vi "BRig_RT__Case_Exp__State_initTrial__v3.vi"(0 "input_dataCurrent":u16[](array[numeric]), 9 "input_dataBlock":u16[][](array[numeric]), 11 "input_dataTrial":u16[][](array[numeric]), 12 "input_dataExp":u16[](array[numeric])) -> (1 "output_iTrial":u16, 2 "output_nTrial":u16, 3 "output_SolenoidReward":bool, 4 "output_dataCurrent":u16[](array[numeric]), 10 "output_dataBlock":u16[][](array[numeric]), 15 "output_dataTrial":u16[][](array[numeric]))   [LabVIEW 2014]
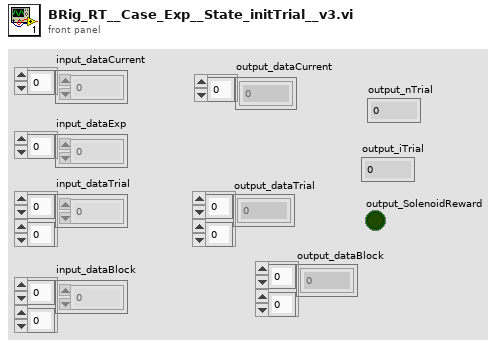
[diagram p1: front panel]
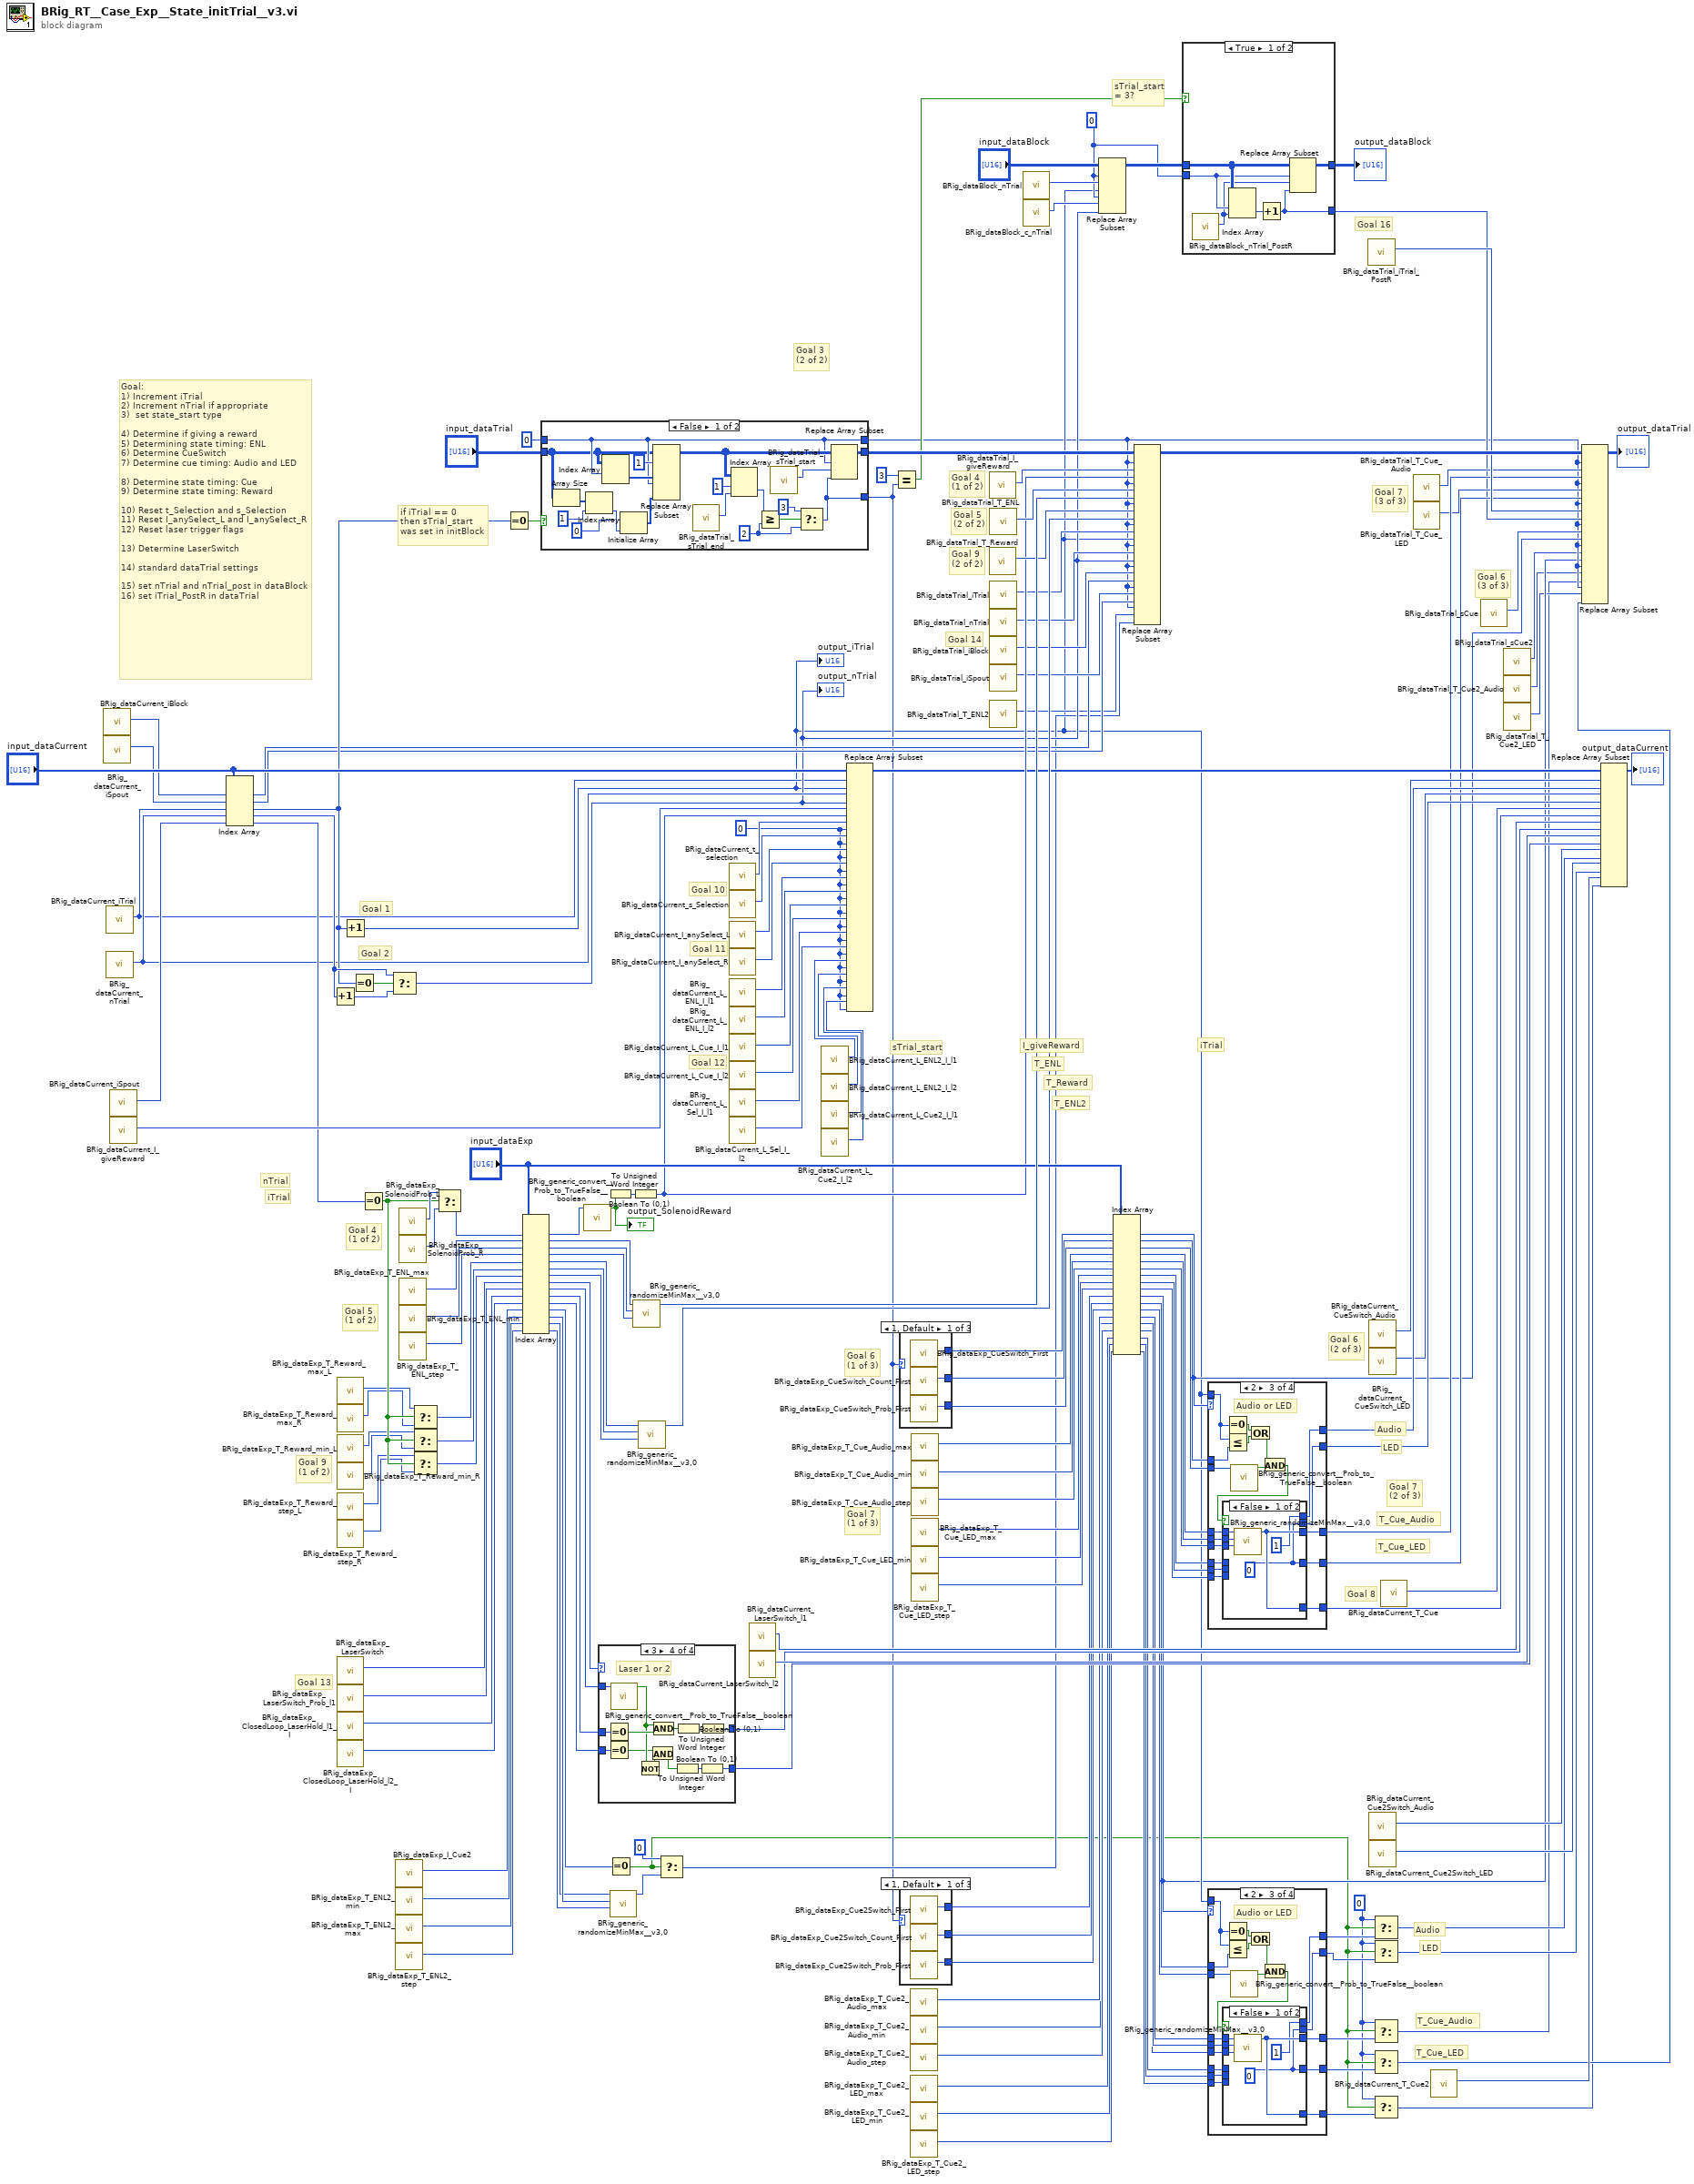
[diagram p0: block diagram]
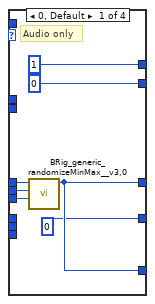
[diagram p2: hidden frame]
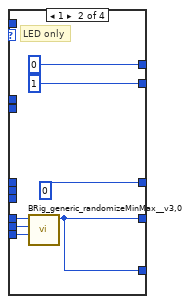
[diagram p3: hidden frame]
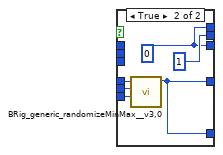
[diagram p4: hidden frame]
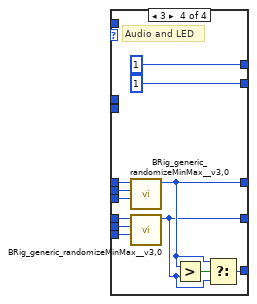
[diagram p5: hidden frame]
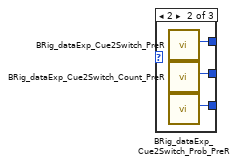
[diagram p6: hidden frame]
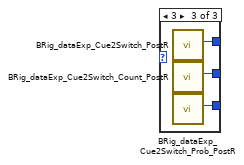
[diagram p7: hidden frame]
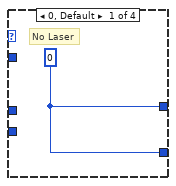
[diagram p9: hidden frame]
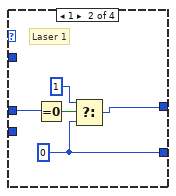
[diagram p10: hidden frame]
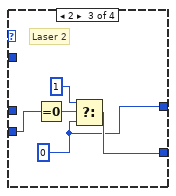
[diagram p11: hidden frame]
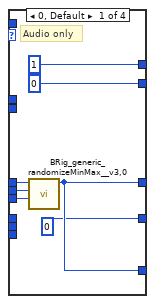
[diagram p12: hidden frame]
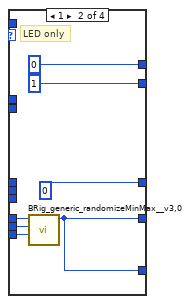
[diagram p13: hidden frame]
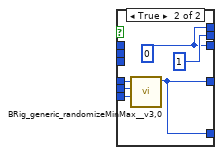
[diagram p14: hidden frame]
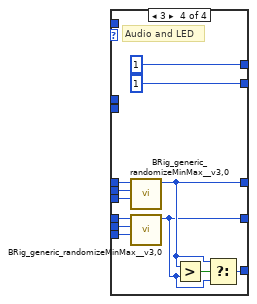
[diagram p15: hidden frame]
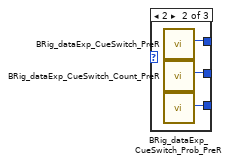
[diagram p16: hidden frame]
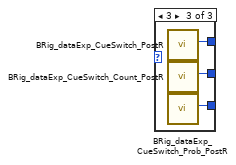
[diagram p17: hidden frame]
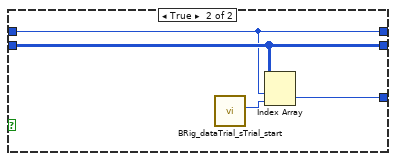
[diagram p18: hidden frame]
diagram:
  w1 = u16 0 ("t")
  w61 = 0 ("disabled index (row)")
  w40 = u16 0 ("new element/subarray")
  # "T_Cue_LED"
  # "T_Cue_Audio"
  # "LED"
  # "Audio"
  # "T_ENL2"
  # "Goal 16"
  # "Goal 6\n(3 of 3)"
  # "iTrial"
  # "sTrial_start\n= 3?"
  # "nTrial"
  # "Goal 14"
  # "Goal 13"
  # "iTrial"
  # "Goal 8"
  # "Goal 7\n(3 of 3)"
  # "Goal 7\n(2 of 3)"
  # "Goal 7\n(1 of 3)"
  # "T_Cue_LED"
  # "T_Cue_Audio"
  # "I_giveReward"
  # "Goal 4\n(1 of 2)"
  # "T_Reward"
  # "Goal 9\n(2 of 2)"
  # "Goal 9\n(1 of 2)"
  # "Goal 12"
  # "Goal 11"
  # "Goal 10"
  # "T_ENL"
  # "sTrial_start"
  # "LED"
  # "Audio"
  # "Goal 6\n(2 of 3)"
  # "Goal 6\n(1 of 3)"
  # "Goal 3\n(2 of 2)"
  # "Goal 5\n(2 of 2)"
  # "Goal 5\n(1 of 2)"
  # "Goal 4\n(1 of 2)"
  # "if iTrial == 0\nthen sTrial_start\nwas set in initBlock"
  # "Goal 2"
  # "Goal 1"
  # "Goal:\n1) Increment iTrial\n2) Increment nTrial if appropriate\n3)  set state_start type\n\n4) Determine if giving a reward\n5) Determining state timing: ENL\n6) Determine CueSwitch\n7) Determine cue timing: Audio and LED\n\n8) Determine state timing: Cue\n9) Determine state timing: Reward\n\n10) Reset t_Selection and s_Selection\n11) Reset I_anySelect_L and I_anySelect_R\n12) Reset laser trigger flags\n\n13) Determine LaserSwitch\n\n14) standard dataTrial settings\n\n15) set nTrial and nTrial_post in dataBlock\n16) set iTrial_PostR in dataTrial"
  n1 = call "BRig_dataCurrent_iBlock.vi"() -> ("output_iBlock"=w78:i32)  [unwired: 11 in]
  n2 = call "BRig_dataCurrent_iSpout.vi"() -> ("output_iSpout"=w77:i32)  [unwired: 11 in]
  n3 = call "BRig_dataCurrent_iTrial.vi"() -> ("output_iTrial"=w57:i32)  [unwired: 11 in]
  n4 = call "BRig_dataCurrent_nTrial.vi"() -> ("output_nTrial"=w59:i32)  [unwired: 11 in]
  n5 = call "BRig_dataCurrent_iSpout.vi"() -> ("output_iSpout"=w69:i32)  [unwired: 11 in]
  n6 = call "BRig_dataCurrent_I_giveReward.vi"() -> ("output_I_giveReward"=w169:i32)  [unwired: 11 in]
  n7 = Index Array(array="input_dataCurrent", index #1=w78, index #2=w77, index #3=w57, index #4=w59, index #5=w69) -> (element #1=w88:u16, element #2=w87:u16, element #3=w101:u16, element #4=w175:u16, element #5=w68:u16)
  n8 = Increment(x=w175) -> (x+1=w174:u16)
  n9 = call "BRig_dataExp_T_Reward_max_L.vi"() -> ("output_T_Reward_max_L"=w134:i32)  [unwired: 11 in]
  n10 = call "BRig_dataExp_T_Reward_max_R.vi"() -> ("output_T_Reward_max_R"=w133:i32)  [unwired: 11 in]
  n11 = call "BRig_dataExp_T_Reward_min_L.vi"() -> ("output_Tcycle_Reward_min_L"=w132:i32)  [unwired: 11 in]
  n12 = call "BRig_dataExp_T_Reward_min_R.vi"() -> ("output_T_Reward_min_R"=w131:i32)  [unwired: 11 in]
  n13 = call "BRig_dataExp_T_Reward_step_L.vi"() -> ("output_T_Reward_step_L"=w130:i32)  [unwired: 11 in]
  n14 = call "BRig_dataExp_T_Reward_step_R.vi"() -> ("output_T_Reward_step_R"=w129:i32)  [unwired: 11 in]
  n15 = call "BRig_dataExp_LaserSwitch.vi"() -> ("output_LaserSwitch"=w100:i32)  [unwired: 11 in]
  n16 = call "BRig_dataExp_LaserSwitch_Prob_l1.vi"() -> ("output_LaserSwitch_Probability_L1"=w99:i32)  [unwired: 11 in]
  n17 = call "BRig_dataExp_ClosedLoop_LaserHold_l1_I.vi"() -> ("output_CloseLoop_LaserHold_l1_I"=w74:i32)  [unwired: 11 in]
  n18 = call "BRig_dataExp_ClosedLoop_LaserHold_l2_I.vi"() -> ("output_CloseLoop_LaserHold_l2_I"=w73:i32)  [unwired: 11 in]
  n19 = Increment(x=w101) -> (x+1=w29:u16)
  "output_iTrial" <- w29
  n20 = Equal To 0?(x=w101) -> (x = 0?=w173:bool)
  n21 = Equal To 0?(x=w68) -> (x = 0?=w135:bool)
  n22 = Select(t=w175, s=w173, f=w174) -> (s? t:f=w58:u16)
  "output_nTrial" <- w58
  n23 = call "BRig_dataExp_I_Cue2.vi"() -> ("output_I_Cue2"=w56:i32)  [unwired: 11 in]
  n24 = call "BRig_dataExp_T_ENL2_min.vi"() -> ("output_T_ENL2_min"=w55:i32)  [unwired: 11 in]
  n25 = call "BRig_dataExp_T_ENL2_max.vi"() -> ("output_T_ENL2_max"=w54:i32)  [unwired: 11 in]
  n26 = call "BRig_dataExp_T_ENL2_step.vi"() -> ("output_T_ENL2_step"=w53:i32)  [unwired: 11 in]
  n27 = call "BRig_dataExp_SolenoidProb_L.vi"() -> ("output_SolenoidProbability_L"=w168:i32)  [unwired: 11 in]
  n28 = call "BRig_dataExp_SolenoidProb_R.vi"() -> ("output_SolenoidProbability_R"=w167:i32)  [unwired: 11 in]
  n29 = call "BRig_dataExp_T_ENL_max.vi"() -> ("output_T_ENL_max"=w161:i32)  [unwired: 11 in]
  n30 = call "BRig_dataExp_T_ENL_min.vi"() -> ("output_T_ENL_min"=w162:i32)  [unwired: 11 in]
  n31 = call "BRig_dataExp_T_ENL_step.vi"() -> ("output_T_ENL_step"=w163:i32)  [unwired: 11 in]
  n32 = Select(t=w134, s=w135, f=w133) -> (s? t:f=w128:i32)
  n33 = Select(t=w132, s=w135, f=w131) -> (s? t:f=w127:i32)
  n34 = Select(t=w130, s=w135, f=w129) -> (s? t:f=w126:i32)
  n35 = Select(t=w168, s=w135, f=w167) -> (s? t:f=w166:i32)
  n36 = Equal To 0?(x=w101) -> (x = 0?=w172:bool)
  n37 = Index Array(array="input_dataExp", index #1=w166, index #2=w161, index #3=w162, index #4=w163, index #5=w128, index #6=w127, index #7=w126, index #8=w100, index #9=w99, index #10=w74, index #11=w73, index #12=w56, index #13=w55, index #14=w54, index #15=w53) -> (element #1=w165:u16, element #2=w160:u16, element #3=w159:u16, element #4=w158:u16, element #5=w125:u16, element #6=w124:u16, element #7=w123:u16, element #8=w98:u16, element #9=w97:u16, element #10=w72:u16, element #11=w71:u16, element #12=w50:u16, element #13=w49:u16, element #14=w48:u16, element #15=w47:u16)
  n38 = case shown="False" w172 {
    tunnel: "input_dataTrial" -> [w182 w199]
    tunnel: [w193 w199] -> w157
    tunnel: 0 -> [w183 w198]
    tunnel: [w183 w198] -> w13
    tunnel: [w189 w196] -> w39
    frame False {
      w190 = u16 2 ("y")
      n39 = Array Size(array=w182) -> (size(s)=w181:i32[])
      n40 = Index Array(array=w181, index=1) -> (element=w179:i32)
      n41 = Index Array(array=w182, index (row)=w183) -> (element=w186:u16[])  [unwired: 1 in]
      n42 = Initialize Array(u16 0 ("index"), w179) -> (w177:u16[])
      n43 = Replace Array Subset(array=w182, new element #1=w186, index (row) #1=1 ("index (row)"), new element #2=w177, index (row) #2=w183) -> (w184:u16[][])  [unwired: 2 in]
      n44 = call "BRig_dataTrial_sTrial_end.vi"() -> ("output_sTrial_end"=w195:i32)  [unwired: 11 in]
      n45 = Index Array(array=w184, index (row)=1 ("disabled index (row)"), index (col)=w195) -> (element=w194:u16)
      n46 = Greater Or Equal?(x=w194, y=w190) -> (x >= y?=w192:bool)
      n47 = call "BRig_dataTrial_sTrial_start.vi"() -> ("output_sTrial_start"=w188:i32)  [unwired: 11 in]
      n48 = Select(t=u16 3 ("y"), s=w192, f=w190) -> (s? t:f=w189:u16)
      n49 = Replace Array Subset(array=w184, new element=w189, index (row)=w183, index (col)=w188) -> (w193:u16[][])
    }
    frame True {
      n50 = call "BRig_dataTrial_sTrial_start.vi"() -> ("output_sTrial_start"=w197:i32)  [unwired: 11 in]
      n51 = Index Array(array=w199, index (row)=w198, index (col)=w197) -> (element=w196:u16)
    }
  }
  n52 = call "BRig_generic_convert__Prob_to_TrueFalse__boolean.vi"("input_probability_u16"=w165) -> ("output_TF"=w164:bool)  [unwired: 10 in]
  "output_SolenoidReward" <- w164
  n53 = case shown="3" w98 {
    tunnel: [w200 w201 w206 w220] -> w95
    tunnel: [w200 w202 w207 w219] -> w94
    tunnel: w97 -> [_ _ _ w223]
    tunnel: w72 -> [_ w205 _ w218]
    tunnel: w71 -> [_ _ w208 w217]
    frame 0, Default {
      w200 = u16 0
      # "No Laser"
    }
    frame 1 {
      w202 = u16 0
      # "Laser 1"
      n54 = Equal To 0?(x=w205) -> (x = 0?=w204:bool)
      n55 = Select(t=u16 1, s=w204, f=w202) -> (s? t:f=w201:u16)
    }
    frame 2 {
      w206 = u16 0
      # "Laser 2"
      n56 = Equal To 0?(x=w208) -> (x = 0?=w210:bool)
      n57 = Select(t=u16 1, s=w210, f=w206) -> (s? t:f=w207:u16)
    }
    frame 3 {
      # "Laser 1 or 2"
      n58 = Equal To 0?(x=w218) -> (x = 0?=w216:bool)
      n59 = Equal To 0?(x=w217) -> (x = 0?=w212:bool)
      n60 = call "BRig_generic_convert__Prob_to_TrueFalse__boolean.vi"("input_probability_u16"=w223) -> ("output_TF"=w215:bool)  [unwired: 10 in]
      n61 = Not(x=w215) -> (.not. x?=w213:bool)
      n62 = And(x=w212, y=w213) -> (x .and. y?=w211:bool)
      n63 = And(x=w215, y=w216) -> (x .and. y?=w214:bool)
      n64 = Boolean To (0,1)(Boolean=w211) -> (0, 1=w222:i16)
      n65 = Boolean To (0,1)(Boolean=w214) -> (0, 1=w221:i16)
      n66 = To Unsigned Word Integer(number=w222) -> (unsigned 16bit integer=w219:u16)
      n67 = To Unsigned Word Integer(number=w221) -> (unsigned 16bit integer=w220:u16)
    }
  }
  n68 = Boolean To (0,1)(Boolean=w164) -> (0, 1=w176:i16)
  n69 = Equal To 0?(x=w50) -> (x = 0?=w2:bool)
  n70 = call "BRig_generic_randomizeMinMax__v3,0.vi"("Input_Increment"=w47, "Input_Min"=w49, "Input_Max"=w48) -> ("Output"=w52:u16)  [unwired: 8 in]
  n71 = To Unsigned Word Integer(number=w176) -> (unsigned 16bit integer=w119:u16)
  n72 = call "BRig_generic_randomizeMinMax__v3,0.vi"("Input_Increment"=w158, "Input_Min"=w159, "Input_Max"=w160) -> ("Output"=w155:u16)  [unwired: 8 in]
  n73 = call "BRig_generic_randomizeMinMax__v3,0.vi"("Input_Increment"=w123, "Input_Min"=w124, "Input_Max"=w125) -> ("Output"=w121:u16)  [unwired: 8 in]
  n74 = Select(t=u16 0, s=w2, f=w52) -> (s? t:f=w45:u16)
  n75 = call "BRig_dataCurrent_t_selection.vi"() -> ("output_t_selection"=w145:i32)  [unwired: 11 in]
  n76 = call "BRig_dataCurrent_s_Selection.vi"() -> ("output_s_Selection"=w144:i32)  [unwired: 11 in]
  n77 = call "BRig_dataCurrent_I_anySelect_L.vi"() -> ("output_IanySelect_L"=w143:i32)  [unwired: 11 in]
  n78 = call "BRig_dataCurrent_I_anySelect_R.vi"() -> ("output_IanySelect_R"=w142:i32)  [unwired: 11 in]
  n79 = call "BRig_dataCurrent_L_ENL_I_l1.vi"() -> ("output_L_ENL_I_l1"=w141:i32)  [unwired: 11 in]
  n80 = call "BRig_dataCurrent_L_ENL_I_l2.vi"() -> ("output_L_ENL_I_l2"=w140:i32)  [unwired: 11 in]
  n81 = call "BRig_dataCurrent_L_Cue_I_l1.vi"() -> ("output_L_Cue_I_l1"=w139:i32)  [unwired: 11 in]
  n82 = call "BRig_dataCurrent_L_Cue_I_l2.vi"() -> ("output_L_Cue_I_l2"=w138:i32)  [unwired: 11 in]
  n83 = call "BRig_dataCurrent_L_Sel_I_l1.vi"() -> ("output_L_Sel_I_l1"=w137:i32)  [unwired: 11 in]
  n84 = call "BRig_dataCurrent_L_Sel_I_l2.vi"() -> ("output_L_Sel_I_l2"=w136:i32)  [unwired: 11 in]
  n85 = call "BRig_dataCurrent_LaserSwitch_l1.vi"() -> ("output_LaserSwitch_l1"=w93:i32)  [unwired: 11 in]
  n86 = call "BRig_dataCurrent_LaserSwitch_l2.vi"() -> ("output_LaserSwitch_l2"=w96:i32)  [unwired: 11 in]
  n87 = call "BRig_dataCurrent_L_ENL2_I_l1.vi"() -> ("output_L_ENL2_I_l1"=w44:i32)  [unwired: 11 in]
  n88 = call "BRig_dataCurrent_L_ENL2_I_l2.vi"() -> ("output_L_ENL2_I_l2"=w43:i32)  [unwired: 11 in]
  n89 = call "BRig_dataCurrent_L_Cue2_I_l1.vi"() -> ("output_L_Cue2_I_l1"=w42:i32)  [unwired: 11 in]
  n90 = call "BRig_dataCurrent_L_Cue2_I_l2.vi"() -> ("output_L_Cue2_I_l2"=w41:i32)  [unwired: 11 in]
  n91 = Replace Array Subset(array="input_dataCurrent", new element #1=w29, index #1=w57, new element #2=w58, index #2=w59, new element #3=w119, index #3=w169, new element #4=w40, index #4=w145, new element #5=w40, index #5=w144, new element #6=w40, index #6=w143, new element #7=w40, index #7=w142, new element #8=w40, index #8=w141, new element #9=w40, index #9=w140, new element #10=w40, index #10=w139, new element #11=w40, index #11=w138, new element #12=w40, index #12=w137, new element #13=w40, index #13=w136, new element #14=w40, index #14=w44, new element #15=w40, index #15=w43, new element #16=w40, index #16=w42, new element #17=w40, index #17=w41) -> (w85:u16[])
  n92 = Equal?(x=u16 3 ("y"), y=w39) -> (x = y?=w62:bool)
  n93 = case shown="1, Default" w39 {
    tunnel: [w226 w227 w232] -> w152
    tunnel: [w225 w228 w231] -> w151
    tunnel: [w224 w229 w230] -> w150
    frame 1, Default {
      n94 = call "BRig_dataExp_CueSwitch_First.vi"() -> ("output_CueSwitch_First"=w226:i32)  [unwired: 11 in]
      n95 = call "BRig_dataExp_CueSwitch_Count_First.vi"() -> ("output_CueSwitch_Count_First"=w225:i32)  [unwired: 11 in]
      n96 = call "BRig_dataExp_CueSwitch_Prob_First.vi"() -> ("output_CueSwitch_Prob_First"=w224:i32)  [unwired: 11 in]
    }
    frame 2 {
      n97 = call "BRig_dataExp_CueSwitch_PreR.vi"() -> ("output_CueSwitch_PreR"=w227:i32)  [unwired: 11 in]
      n98 = call "BRig_dataExp_CueSwitch_Count_PreR.vi"() -> ("output_CueSwitch_Count_PreR"=w228:i32)  [unwired: 11 in]
      n99 = call "BRig_dataExp_CueSwitch_Prob_PreR.vi"() -> ("output_CueSwitch_Prob_PreR"=w229:i32)  [unwired: 11 in]
    }
    frame 3 {
      n100 = call "BRig_dataExp_CueSwitch_PostR.vi"() -> ("output_CueSwitch_PostR"=w232:i32)  [unwired: 11 in]
      n101 = call "BRig_dataExp_CueSwitch_Count_PostR.vi"() -> ("output_CueSwitch_Count_PostR"=w231:i32)  [unwired: 11 in]
      n102 = call "BRig_dataExp_CueSwitch_Prob_PostR.vi"() -> ("output_CueSwitch_Prob_PostR"=w230:i32)  [unwired: 11 in]
    }
  }
  n103 = case shown="1, Default" w39 {
    tunnel: [w235 w238 w241] -> w38
    tunnel: [w234 w237 w240] -> w37
    tunnel: [w233 w236 w239] -> w36
    frame 1, Default {
      n104 = call "BRig_dataExp_Cue2Switch_First.vi"() -> ("output_Cue2Switch_First"=w235:i32)  [unwired: 11 in]
      n105 = call "BRig_dataExp_Cue2Switch_Count_First.vi"() -> ("output_Cue2Switch_Count_First"=w234:i32)  [unwired: 11 in]
      n106 = call "BRig_dataExp_Cue2Switch_Prob_First.vi"() -> ("output_Cue2Switch_Prob_First"=w233:i32)  [unwired: 11 in]
    }
    frame 2 {
      n107 = call "BRig_dataExp_Cue2Switch_PreR.vi"() -> ("output_Cue2Switch_PreR"=w238:i32)  [unwired: 11 in]
      n108 = call "BRig_dataExp_Cue2Switch_Count_PreR.vi"() -> ("output_Cue2Switch_Count_PreR"=w237:i32)  [unwired: 11 in]
      n109 = call "BRig_dataExp_Cue2Switch_Prob_PreR.vi"() -> ("output_Cue2Switch_Prob_PreR"=w236:i32)  [unwired: 11 in]
    }
    frame 3 {
      n110 = call "BRig_dataExp_Cue2Switch_PostR.vi"() -> ("output_Cue2Switch_PostR"=w241:i32)  [unwired: 11 in]
      n111 = call "BRig_dataExp_Cue2Switch_Count_PostR.vi"() -> ("output_Cue2Switch_Count_PostR"=w240:i32)  [unwired: 11 in]
      n112 = call "BRig_dataExp_Cue2Switch_Prob_PostR.vi"() -> ("output_Cue2Switch_Prob_PostR"=w239:i32)  [unwired: 11 in]
    }
  }
  n113 = call "BRig_dataExp_T_Cue2_Audio_max.vi"() -> ("output_T_Cue2_Audio_max"=w35:i32)  [unwired: 11 in]
  n114 = call "BRig_dataExp_T_Cue2_Audio_min.vi"() -> ("output_T_Cue2_Audio_min"=w34:i32)  [unwired: 11 in]
  n115 = call "BRig_dataExp_T_Cue2_Audio_step.vi"() -> ("output_T_Cue2_Audio_step"=w33:i32)  [unwired: 11 in]
  n116 = call "BRig_dataExp_T_Cue2_LED_max.vi"() -> ("output_T_Cue2_LED_max"=w32:i32)  [unwired: 11 in]
  n117 = call "BRig_dataExp_T_Cue2_LED_min.vi"() -> ("output_T_Cue2_LED_min"=w31:i32)  [unwired: 11 in]
  n118 = call "BRig_dataExp_T_Cue2_LED_step.vi"() -> ("output_T_Cue2_LED_step"=w30:i32)  [unwired: 11 in]
  n119 = call "BRig_dataExp_T_Cue_Audio_max.vi"() -> ("output_T_Cue_Audio_max"=w118:i32)  [unwired: 11 in]
  n120 = call "BRig_dataExp_T_Cue_Audio_min.vi"() -> ("output_T_Cue_Audio_min"=w117:i32)  [unwired: 11 in]
  n121 = call "BRig_dataExp_T_Cue_Audio_step.vi"() -> ("output_T_Cue_Audio_step"=w116:i32)  [unwired: 11 in]
  n122 = call "BRig_dataExp_T_Cue_LED_max.vi"() -> ("output_T_Cue_LED_max"=w115:i32)  [unwired: 11 in]
  n123 = call "BRig_dataExp_T_Cue_LED_min.vi"() -> ("output_T_Cue_LED_min"=w114:i32)  [unwired: 11 in]
  n124 = call "BRig_dataExp_T_Cue_LED_step.vi"() -> ("output_T_Cue_LED_step"=w113:i32)  [unwired: 11 in]
  n125 = call "BRig_dataTrial_I_giveReward.vi"() -> ("output_I_giveReward"=w120:i32)  [unwired: 11 in]
  n126 = call "BRig_dataTrial_T_Reward.vi"() -> ("output_T_Reward"=w122:i32)  [unwired: 11 in]
  n127 = call "BRig_dataTrial_T_ENL.vi"() -> ("output_T_ENL"=w156:i32)  [unwired: 11 in]
  n128 = call "BRig_dataTrial_iTrial.vi"() -> ("output_iTrial"=w92:i32)  [unwired: 11 in]
  n129 = call "BRig_dataTrial_nTrial.vi"() -> ("output_nTrial"=w91:i32)  [unwired: 11 in]
  n130 = call "BRig_dataTrial_iBlock.vi"() -> ("output_iBlock"=w90:i32)  [unwired: 11 in]
  n131 = call "BRig_dataTrial_iSpout.vi"() -> ("output_iSpout"=w89:i32)  [unwired: 11 in]
  n132 = call "BRig_dataTrial_T_ENL2.vi"() -> ("output_T_ENL2"=w46:i32)  [unwired: 11 in]
  n133 = call "BRig_dataBlock_nTrial.vi"() -> ("output_nTrial"=w64:i32)  [unwired: 11 in]
  n134 = call "BRig_dataBlock_c_nTrial.vi"() -> ("output_c_nTrial"=w63:i32)  [unwired: 11 in]
  n135 = Replace Array Subset(array="input_dataBlock", new element #1=w29, index (row) #1=w61, index (col) #1=w64, new element #2=w58, index (row) #2=w61, index (col) #2=w63) -> (w65:u16[][])
  n136 = Index Array(array="input_dataExp", index #1=w152, index #2=w151, index #3=w150, index #4=w118, index #5=w117, index #6=w116, index #7=w115, index #8=w114, index #9=w113, index #10=w38, index #11=w37, index #12=w36, index #13=w35, index #14=w34, index #15=w33, index #16=w32, index #17=w31, index #18=w30) -> (element #1=w75:u16, element #2=w112:u16, element #3=w111:u16, element #4=w110:u16, element #5=w109:u16, element #6=w108:u16, element #7=w107:u16, element #8=w106:u16, element #9=w105:u16, element #10=w12:u16, element #11=w28:u16, element #12=w27:u16, element #13=w26:u16, element #14=w25:u16, element #15=w24:u16, element #16=w23:u16, element #17=w22:u16, element #18=w21:u16)
  n137 = Replace Array Subset(array=w157, new element #1=w119, index (row) #1=w13, index (col) #1=w120, new element #2=w155, index (row) #2=w13, index (col) #2=w156, new element #3=w121, index (row) #3=w13, index (col) #3=w122, new element #4=w29, index (row) #4=w13, index (col) #4=w92, new element #5=w58, index (row) #5=w13, index (col) #5=w91, new element #6=w88, index (row) #6=w13, index (col) #6=w90, new element #7=w87, index (row) #7=w13, index (col) #7=w89, new element #8=w45, index (row) #8=w13, index (col) #8=w46) -> (w84:u16[][])
  n138 = case shown="True" w62 {
    tunnel: w65 -> [w247 w248]
    tunnel: [w245 w248] -> w86
    tunnel: [w242 _] -> w60
    tunnel: w61 -> [w244 _]
    frame True {
      n139 = call "BRig_dataBlock_nTrial_PostR.vi"() -> ("output_nTrial_PostR"=w243:i32)  [unwired: 11 in]
      n140 = Index Array(array=w247, index (row)=w244, index (col)=w243) -> (element=w246:u16)
      n141 = Increment(x=w246) -> (x+1=w242:u16)
      n142 = Replace Array Subset(array=w247, new element=w242, index (row)=w244, index (col)=w243) -> (w245:u16[][])
    }
    frame False {
    }
  }
  "output_dataBlock" <- w86
  n143 = case shown="2" w75 {
    tunnel: [u16 1 u16 0 w267 u16 1] -> w148
    tunnel: [u16 0 u16 1 w266 u16 1] -> w146
    tunnel: w112 -> [_ _ w280 _]
    tunnel: w111 -> [_ _ w277 _]
    tunnel: w110 -> [w253 _ w273 w303]
    tunnel: w109 -> [w252 _ w272 w302]
    tunnel: w108 -> [w251 _ w271 w301]
    tunnel: w107 -> [_ w260 w265 w300]
    tunnel: w106 -> [_ w259 w264 w299]
    tunnel: w105 -> [_ w258 w263 w298]
    tunnel: [w250 u16 0 ("Output") w270 w296] -> w82
    tunnel: [u16 0 ("Output") w257 w268 w295] -> w81
    tunnel: [w250 w257 w269 w294] -> w102
    tunnel: w29 -> [_ _ w281 _]
    frame 0, Default {
      # "Audio only"
      n144 = call "BRig_generic_randomizeMinMax__v3,0.vi"("Input_Increment"=w251, "Input_Min"=w252, "Input_Max"=w253) -> ("Output"=w250:u16)  [unwired: 8 in]
    }
    frame 1 {
      # "LED only"
      n145 = call "BRig_generic_randomizeMinMax__v3,0.vi"("Input_Increment"=w258, "Input_Min"=w259, "Input_Max"=w260) -> ("Output"=w257:u16)  [unwired: 8 in]
    }
    frame 2 {
      # "Audio or LED"
      n146 = Equal To 0?(x=w281) -> (x = 0?=w279:bool)
      n147 = Less Or Equal?(x=w281, y=w280) -> (x <= y?=w278:bool)
      n148 = call "BRig_generic_convert__Prob_to_TrueFalse__boolean.vi"("input_probability_u16"=w277) -> ("output_TF"=w276:bool)  [unwired: 10 in]
      n149 = Or(x=w279, y=w278) -> (x .or. y?=w275:bool)
      n150 = And(x=w275, y=w276) -> (x .and. y?=w274:bool)
      n151 = case shown="False" w274 {
        tunnel: w273 -> [w287 _]
        tunnel: w272 -> [w286 _]
        tunnel: w271 -> [w285 _]
        tunnel: [w284 w288] -> w270
        tunnel: [w284 w290] -> w269
        tunnel: [w282 w290] -> w268
        tunnel: [u16 1 w288] -> w267
        tunnel: [w282 u16 1] -> w266
        tunnel: w265 -> [_ w293]
        tunnel: w264 -> [_ w292]
        tunnel: w263 -> [_ w291]
        frame False {
          w282 = u16 0
          n152 = call "BRig_generic_randomizeMinMax__v3,0.vi"("Input_Increment"=w285, "Input_Min"=w286, "Input_Max"=w287) -> ("Output"=w284:u16)  [unwired: 8 in]
        }
        frame True {
          w288 = u16 0
          n153 = call "BRig_generic_randomizeMinMax__v3,0.vi"("Input_Increment"=w291, "Input_Min"=w292, "Input_Max"=w293) -> ("Output"=w290:u16)  [unwired: 8 in]
        }
      }
    }
    frame 3 {
      # "Audio and LED"
      n154 = call "BRig_generic_randomizeMinMax__v3,0.vi"("Input_Increment"=w301, "Input_Min"=w302, "Input_Max"=w303) -> ("Output"=w296:u16)  [unwired: 8 in]
      n155 = call "BRig_generic_randomizeMinMax__v3,0.vi"("Input_Increment"=w298, "Input_Min"=w299, "Input_Max"=w300) -> ("Output"=w295:u16)  [unwired: 8 in]
      n156 = Greater?(x=w296, y=w295) -> (0:w297:bool)
      n157 = Select(t=w296, s=w297, f=w295) -> (s? t:f=w294:u16)
    }
  }
  n158 = case shown="2" w12 {
    tunnel: [u16 1 u16 0 w324 u16 1] -> w19
    tunnel: [u16 0 u16 1 w323 u16 1] -> w20
    tunnel: w28 -> [_ _ w337 _]
    tunnel: w27 -> [_ _ w334 _]
    tunnel: w26 -> [w310 _ w330 w360]
    tunnel: w25 -> [w309 _ w329 w359]
    tunnel: w24 -> [w308 _ w328 w358]
    tunnel: w23 -> [_ w317 w322 w357]
    tunnel: w22 -> [_ w316 w321 w356]
    tunnel: w21 -> [_ w315 w320 w355]
    tunnel: [w307 u16 0 ("Output") w327 w353] -> w8
    tunnel: [u16 0 ("Output") w314 w325 w352] -> w6
    tunnel: [w307 w314 w326 w351] -> w4
    tunnel: w29 -> [_ _ w338 _]
    frame 0, Default {
      # "Audio only"
      n159 = call "BRig_generic_randomizeMinMax__v3,0.vi"("Input_Increment"=w308, "Input_Min"=w309, "Input_Max"=w310) -> ("Output"=w307:u16)  [unwired: 8 in]
    }
    frame 1 {
      # "LED only"
      n160 = call "BRig_generic_randomizeMinMax__v3,0.vi"("Input_Increment"=w315, "Input_Min"=w316, "Input_Max"=w317) -> ("Output"=w314:u16)  [unwired: 8 in]
    }
    frame 2 {
      # "Audio or LED"
      n161 = Equal To 0?(x=w338) -> (x = 0?=w336:bool)
      n162 = Less Or Equal?(x=w338, y=w337) -> (x <= y?=w335:bool)
      n163 = call "BRig_generic_convert__Prob_to_TrueFalse__boolean.vi"("input_probability_u16"=w334) -> ("output_TF"=w333:bool)  [unwired: 10 in]
      n164 = Or(x=w336, y=w335) -> (x .or. y?=w332:bool)
      n165 = And(x=w332, y=w333) -> (x .and. y?=w331:bool)
      n166 = case shown="False" w331 {
        tunnel: w330 -> [w344 _]
        tunnel: w329 -> [w343 _]
        tunnel: w328 -> [w342 _]
        tunnel: [w341 w345] -> w327
        tunnel: [w341 w347] -> w326
        tunnel: [w339 w347] -> w325
        tunnel: [u16 1 w345] -> w324
        tunnel: [w339 u16 1] -> w323
        tunnel: w322 -> [_ w350]
        tunnel: w321 -> [_ w349]
        tunnel: w320 -> [_ w348]
        frame False {
          w339 = u16 0
          n167 = call "BRig_generic_randomizeMinMax__v3,0.vi"("Input_Increment"=w342, "Input_Min"=w343, "Input_Max"=w344) -> ("Output"=w341:u16)  [unwired: 8 in]
        }
        frame True {
          w345 = u16 0
          n168 = call "BRig_generic_randomizeMinMax__v3,0.vi"("Input_Increment"=w348, "Input_Min"=w349, "Input_Max"=w350) -> ("Output"=w347:u16)  [unwired: 8 in]
        }
      }
    }
    frame 3 {
      # "Audio and LED"
      n169 = call "BRig_generic_randomizeMinMax__v3,0.vi"("Input_Increment"=w358, "Input_Min"=w359, "Input_Max"=w360) -> ("Output"=w353:u16)  [unwired: 8 in]
      n170 = call "BRig_generic_randomizeMinMax__v3,0.vi"("Input_Increment"=w355, "Input_Min"=w356, "Input_Max"=w357) -> ("Output"=w352:u16)  [unwired: 8 in]
      n171 = Greater?(x=w353, y=w352) -> (0:w354:bool)
      n172 = Select(t=w353, s=w354, f=w352) -> (s? t:f=w351:u16)
    }
  }
  n173 = call "BRig_dataTrial_iTrial_PostR.vi"() -> ("output_iTrial_PostR"=w83:i32)  [unwired: 11 in]
  n174 = call "BRig_dataCurrent_CueSwitch_Audio.vi"() -> ("output_CueSwitch_Audio"=w149:i32)  [unwired: 11 in]
  n175 = call "BRig_dataCurrent_CueSwitch_LED.vi"() -> ("output_CueSwitch_LED"=w147:i32)  [unwired: 11 in]
  n176 = call "BRig_dataCurrent_Cue2Switch_Audio.vi"() -> ("output_Cue2Switch_Audio"=w18:i32)  [unwired: 11 in]
  n177 = call "BRig_dataCurrent_Cue2Switch_LED.vi"() -> ("output_Cue2Switch_LED"=w17:i32)  [unwired: 11 in]
  n178 = Select(t=w1, s=w2, f=w19) -> (s? t:f=w16:u16)
  n179 = Select(t=w1, s=w2, f=w20) -> (s? t:f=w15:u16)
  n180 = Select(t=w1, s=w2, f=w8) -> (s? t:f=w7:u16)
  n181 = Select(t=w1, s=w2, f=w6) -> (s? t:f=w5:u16)
  n182 = Select(t=w1, s=w2, f=w4) -> (s? t:f=w3:u16)
  n183 = call "BRig_dataCurrent_T_Cue.vi"() -> ("output_T_Cue"=w103:i32)  [unwired: 11 in]
  n184 = call "BRig_dataTrial_T_Cue_Audio.vi"() -> ("output_T_Cue_Audio"=w80:i32)  [unwired: 11 in]
  n185 = call "BRig_dataTrial_T_Cue_LED.vi"() -> ("output_T_Cue_LED"=w79:i32)  [unwired: 11 in]
  n186 = call "BRig_dataCurrent_T_Cue2.vi"() -> ("output_T_Cue2"=w14:i32)  [unwired: 11 in]
  n187 = call "BRig_dataTrial_sCue.vi"() -> ("output_sCue"=w76:i32)  [unwired: 11 in]
  n188 = call "BRig_dataTrial_sCue2.vi"() -> ("output_sCue2"=w11:i32)  [unwired: 11 in]
  n189 = call "BRig_dataTrial_T_Cue2_Audio.vi"() -> ("output_T_Cue2_Audio"=w10:i32)  [unwired: 11 in]
  n190 = call "BRig_dataTrial_T_Cue2_LED.vi"() -> ("output_T_Cue2_LED"=w9:i32)  [unwired: 11 in]
  n191 = Replace Array Subset(array=w84, new element #1=w82, index (row) #1=w13, index (col) #1=w80, new element #2=w81, index (row) #2=w13, index (col) #2=w79, new element #3=w60, index (row) #3=w13, index (col) #3=w83, new element #4=w75, index (row) #4=w13, index (col) #4=w76, new element #5=w12, index (row) #5=w13, index (col) #5=w11, new element #6=w7, index (row) #6=w13, index (col) #6=w10, new element #7=w5, index (row) #7=w13, index (col) #7=w9) -> (→"output_dataTrial":u16[][])
  n192 = Replace Array Subset(array=w85, new element #1=w148, index #1=w149, new element #2=w146, index #2=w147, new element #3=w102, index #3=w103, new element #4=w95, index #4=w93, new element #5=w94, index #5=w96, new element #6=w16, index #6=w18, new element #7=w15, index #7=w17, new element #8=w3, index #8=w14) -> (→"output_dataCurrent":u16[])
